vi "Unit Test empty class layer.vi"() -> ()   [LabVIEW 2019, in "Sports Unit Tests.lvclass"]
uses:
  Sports Unit Tests.lvclass
  Classes/Pele/Pele.lvclass
  C:/DSCE code/Serialization/blueserializationdemo/Test/Sports/Classes/Human/Human.lvclass
  C:/DSCE code/Serialization/blueserializationdemo/Test/Sports/Classes/Sports Player/Sports Player.lvclass
  Classes/Human/Human.lvclass/Human.ctl
  Classes/Sports Player/Sports Player.lvclass/Sports Player.ctl
  Classes/Pele/Pele.lvclass/Pele.ctl
  Classes/Human/Write Age (years).vi
  Classes/Human/Write alive_.vi
  Classes/Human/Write Height (ft).vi
  Classes/Human/Write Name.vi
  Classes/Sports Player/Write Earnings (dollars).vi
  Classes/Sports Player/Write Professional_.vi
  Classes/Sports Player/Write Sponsor.vi
  Classes/Pele/Write Nickname.vi
  <vilib>/Utility/error.llb/Clear Errors.vi
  <vilib>/addons/_JKI Toolkits/Caraya/classes/Test/Define Test.vi
  <vilib>/addons/_JKI Toolkits/Caraya/classes/Assert/Assert Equal Value_Variant.vi
  <vilib>/addons/_JKI Toolkits/Caraya/classes/Assert/Assert Not Error.vi
  <vilib>/addons/_JKI Toolkits/Caraya/classes/Assert/Assert.lvclass
  <userlib>/Blue Origin/BlueSerialization/BlueSerializer/BlueSerializer.lvclass
panel:
  out "Table":string[][](table)
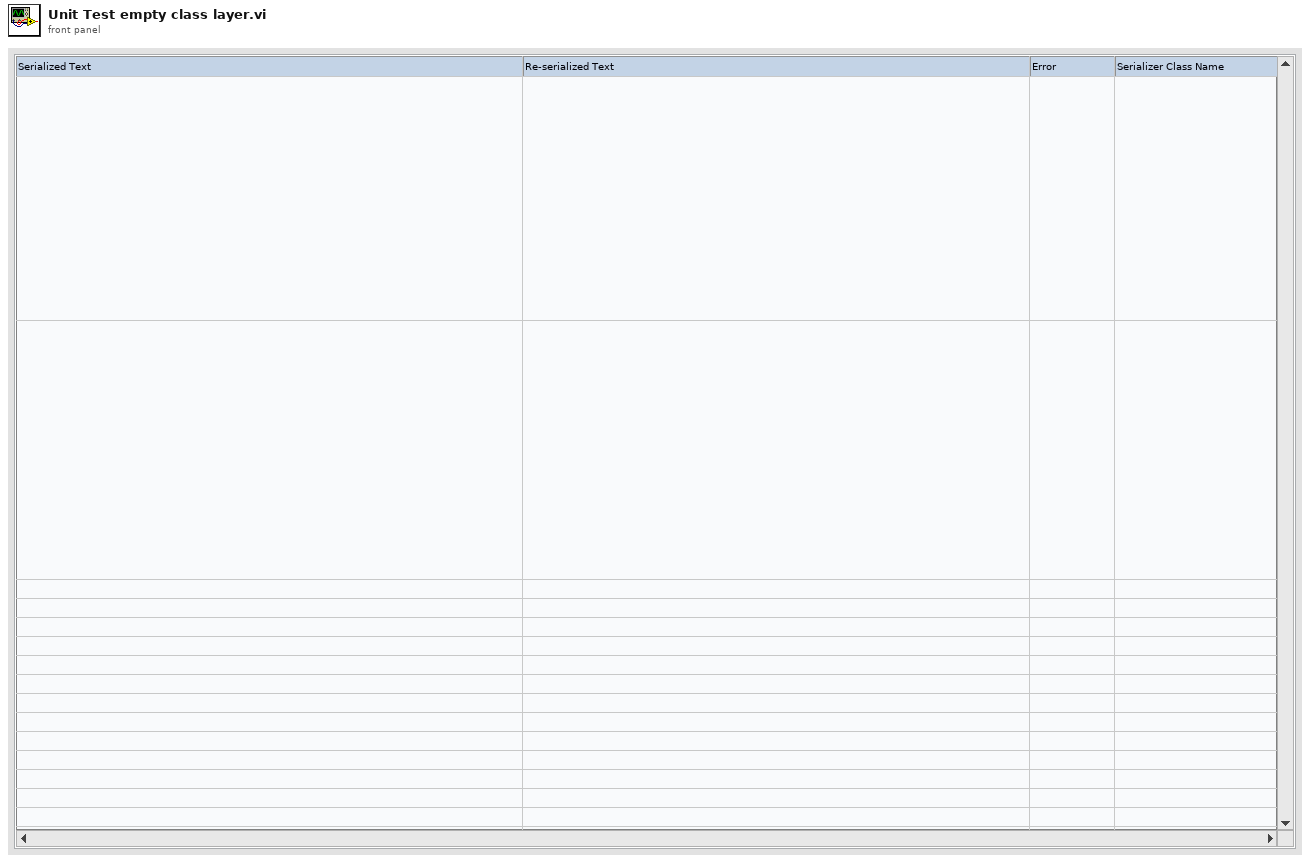
[diagram p1: front panel]
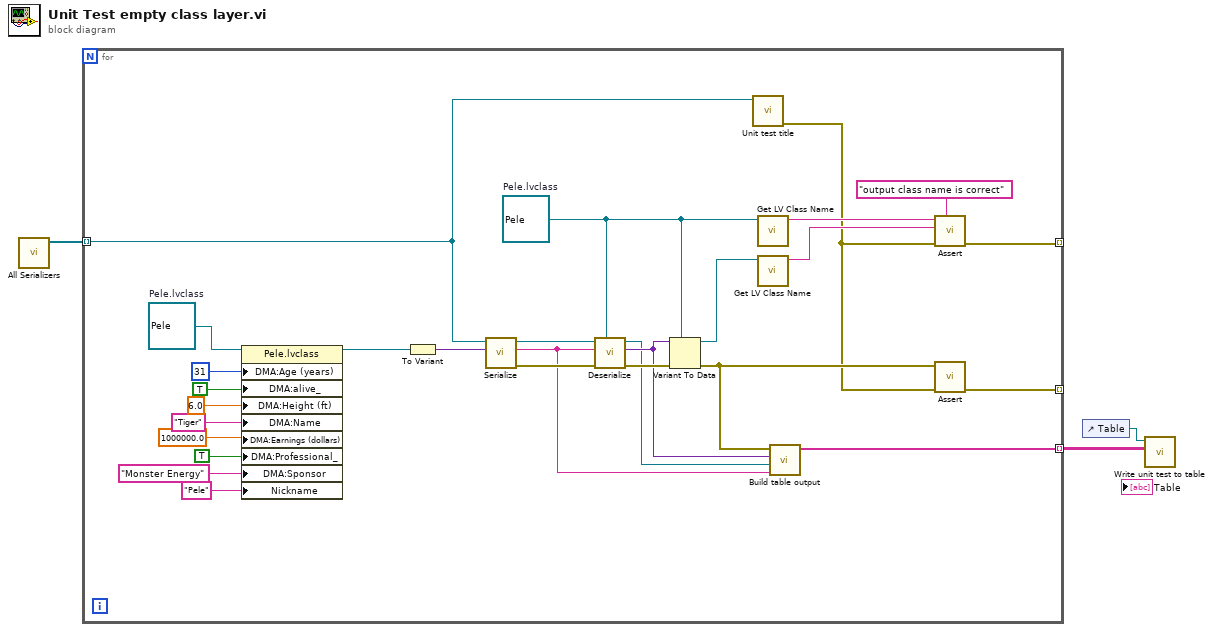
[diagram p0: block diagram]
diagram:
  n1 = call "All Serializers.vi"() -> ("All serializers"=w2:refnum<class "BlueSerializer.lvclass">[])  [unwired: 11 in]
  n2 = for {
    tunnel: w2 -> [w10] mode=indexing
    tunnel: [w15] -> _ mode=indexing
    tunnel: [w11] -> w1 mode=indexing
    tunnel: [w5] -> _ mode=indexing
    w4 = refnum<class "Pele.lvclass"> refnum  # Pele.lvclass
    w9 = refnum<class "Pele.lvclass"> refnum  # Pele.lvclass
    n3 = property on="Property Node" class="Pele.lvclass"(reference=w9, "DMA:Age (years)"=u16 31 ("Age (years)"), "DMA:alive_"=TRUE ("alive_"), "DMA:Height (ft)"=6.0 ("Height (ft)"), "DMA:Name"="Tiger" ("Name"), "DMA:Earnings (dollars)"=1000000.0 ("Earnings (dollars)"), "DMA:Professional_"=TRUE ("Professional_"), "DMA:Sponsor"="Monster Energy" ("Sponsor"), "Nickname"="Pele") -> (reference out=w16:refnum<class "Pele.lvclass">)  [unwired: 1 in, 1 out]
    n4 = To Variant(anything=w16) -> (Variant=w29:variant)
    n5 = call <userlib>:"Serialize.vi"("Anything"=w29, "BlueSerializer in"=w10) -> ("error out"=w31:errorcluster, "Serialized Text"=w12:string, "BlueSerializer out"=w30:refnum<class "BlueSerializer.lvclass">)  [unwired: 7 in]
    n6 = call <userlib>:"Deserialize.vi"("Anything"=w4, "error in (no error)"=w31, "Serialized Text"=w12, "BlueSerializer in"=w30) -> ("error out"=w28:errorcluster, "Variant"=w14:variant, "BlueSerializer out"=w13:refnum<class "BlueSerializer.lvclass">)  [unwired: 5 in]
    n7 = Variant To Data(error in=w28, type=w4, Variant=w14) -> (data=w27:refnum<class "Pele.lvclass">, error out=w7:errorcluster)
    n8 = call "Unit test title.vi"("serializer"=w10) -> ("error out"=w6:errorcluster)  [unwired: 9 in, 1 out]
    n9 = call <vilib>:"Get LV Class Name.vi"("object"=w4) -> ("class name"=w26:string)  [unwired: 9 in, 1 out]
    n10 = call <vilib>:"Get LV Class Name.vi"("object"=w27) -> ("class name"=w25:string)  [unwired: 9 in, 1 out]
    n11 = call "Build table output.vi"("serialized text"=w12, "BlueSerializer in"=w13, "deserialized variant"=w14, "variant to data error"=w7) -> ("table output"=w11:string[])  [unwired: 7 in]
    n12 = call-poly <vilib>:"Assert.vi"("Label"="output class name is correct", "error in (no error)"=w6, "Y"=w25, "X"=w26) -> ("error out"=w15:errorcluster)  [unwired: 7 in]
    n13 = call-poly <vilib>:"Assert.vi"("error in (no error)"=w6, "Not Error?"=w7) -> ("error out"=w5:errorcluster)  [unwired: 9 in]
  }
  n14 = control-ref of="Table"() -> (w3:refnum<vi>)
  n15 = call "Write unit test to table.vi"("Table"=w1, "Table ref in"=w3) -> ()  [unwired: 9 in, 1 out]
